vi "Pay.vi"(8 "error in (no error)":errorcluster, 10 "IDepositable":refnum<class "IDepositable.lvclass">, 11 "IIncome in":refnum<class "IIncome.lvclass">) -> (0 "error out":errorcluster, 3 "IIncome out":refnum<class "IIncome.lvclass">)   [LabVIEW 2020, in "IIncome.lvclass"]
uses:
  IIncome.lvclass
  IDepositable/IDepositable.lvclass
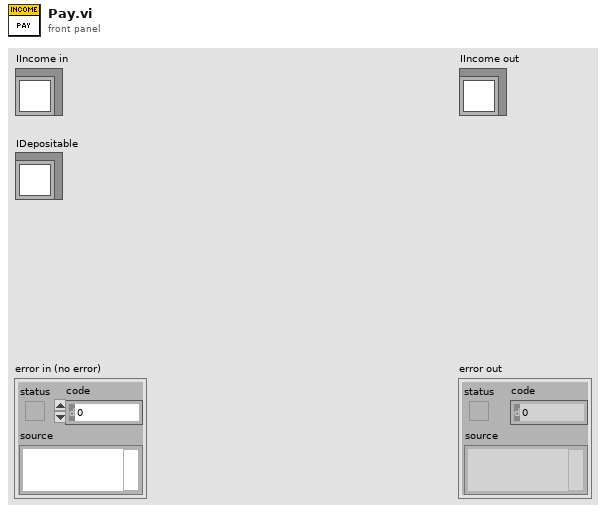
[diagram p1: front panel]
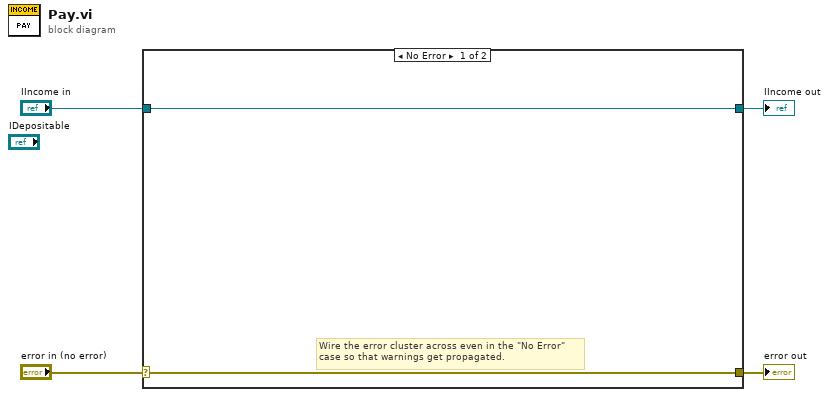
[diagram p0: block diagram]
diagram:
  n1 = case shown="No Error" "error in (no error)" {
    selector: "error in (no error)" -> [w5 w8]
    tunnel: [w5 w8] -> w3
    tunnel: [w6 w7] -> w1
    tunnel: "IIncome in" -> [w6 w7]
    frame No Error {
      # "Wire the error cluster across even in the \"No Error\"\ncase so that warnings get propagated."
    }
    frame Error {
    }
  }
  "error out" <- w3
  "IIncome out" <- w1
